vi "Count Encoder.vi"(0 "Encoder A Prev. Signal In":bool, 5 "Encoder B Prev. Signal In":bool, 7 "Encoder A Signal In":bool, 9 "Encoder B Signal In":bool, 11 "Encoder Count In":i64) -> (15 "Encoder Count Out":i64)   [LabVIEW 2016]
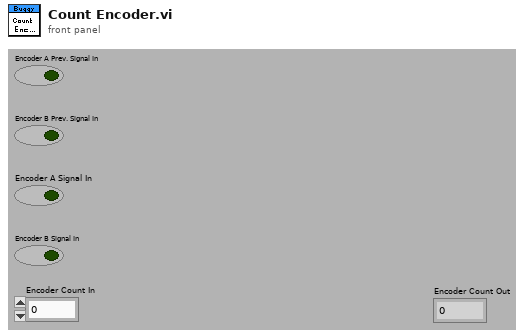
[diagram p1: front panel]
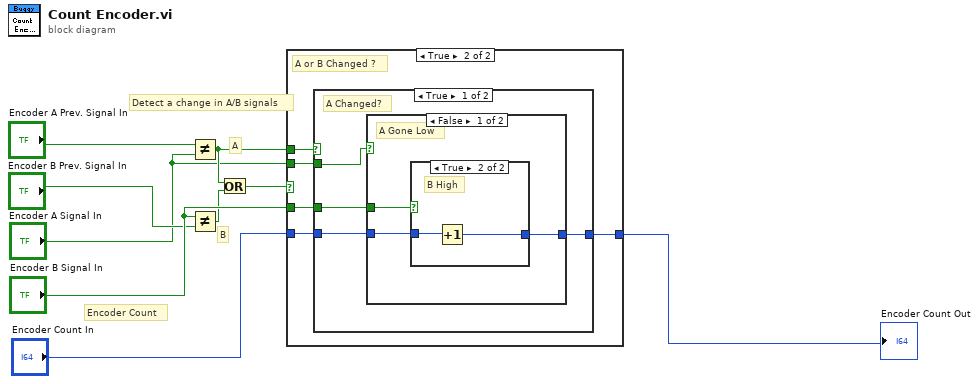
[diagram p0: block diagram]
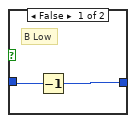
[diagram p3: hidden frame]
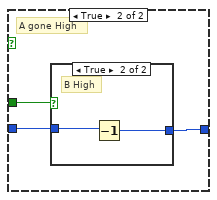
[diagram p4: hidden frame]
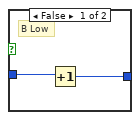
[diagram p5: hidden frame]
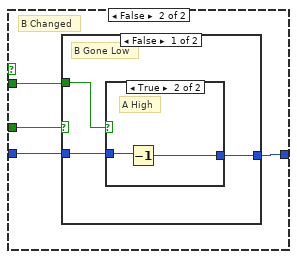
[diagram p6: hidden frame]
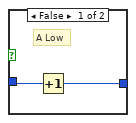
[diagram p7: hidden frame]
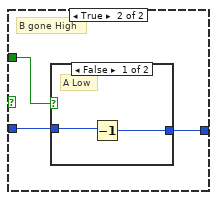
[diagram p8: hidden frame]
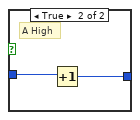
[diagram p9: hidden frame]
diagram:
  # "Encoder Count"
  # "B"
  # "A"
  # "Detect a change in A/B signals"
  n1 = Not Equal?(x="Encoder A Prev. Signal In", y="Encoder A Signal In") -> (x != y?=w8:bool)
  n2 = Not Equal?(x="Encoder B Signal In", y="Encoder B Prev. Signal In") -> (x != y?=w6:bool)
  n3 = Or(x=w8, y=w6) -> (x .or. y?=w5:bool)
  n4 = case shown="True" w5 {
    tunnel: w8 -> [_ w15]
    tunnel: "Encoder Count In" -> [w10 w14]
    tunnel: "Encoder A Signal In" -> [_ w13]
    tunnel: "Encoder B Signal In" -> [_ w12]
    tunnel: [w10 w11] -> w7
    frame False {
      # "A or B not changed Keep Existing encoder count"
    }
    frame True {
      # "A or B Changed ?"
      n5 = case shown="True" w15 {
        tunnel: w14 -> [w19 w37]
        tunnel: w12 -> [w18 w36]
        tunnel: w13 -> [w17 w35]
        tunnel: [w16 w34] -> w11
        frame True {
          # "A Changed?"
          n6 = case shown="False" w17 {
            tunnel: w19 -> [w21 w28]
            tunnel: w18 -> [w22 w29]
            tunnel: [w20 w27] -> w16
            frame False {
              # "A Gone Low"
              n7 = case shown="True" w22 {
                tunnel: w21 -> [w24 w26]
                tunnel: [w23 w25] -> w20
                frame False {
                  # "B Low"
                  n8 = Decrement(x=w24) -> (x-1=w23:i64)
                }
                frame True {
                  # "B High"
                  n9 = Increment(x=w26) -> (x+1=w25:i64)
                }
              }
            }
            frame True {
              # "A gone High"
              n10 = case shown="True" w29 {
                tunnel: w28 -> [w30 w33]
                tunnel: [w31 w32] -> w27
                frame False {
                  # "B Low"
                  n11 = Increment(x=w30) -> (x+1=w31:i64)
                }
                frame True {
                  # "B High"
                  n12 = Decrement(x=w33) -> (x-1=w32:i64)
                }
              }
            }
          }
        }
        frame False {
          # "B Changed"
          n13 = case shown="False" w36 {
            tunnel: w37 -> [w40 w47]
            tunnel: [w39 w46] -> w34
            tunnel: w35 -> [w38 w45]
            frame False {
              # "B Gone Low"
              n14 = case shown="True" w38 {
                tunnel: w40 -> [w42 w44]
                tunnel: [w41 w43] -> w39
                frame False {
                  # "A Low"
                  n15 = Increment(x=w42) -> (x+1=w41:i64)
                }
                frame True {
                  # "A High"
                  n16 = Decrement(x=w44) -> (x-1=w43:i64)
                }
              }
            }
            frame True {
              # "B gone High"
              n17 = case shown="False" w45 {
                tunnel: w47 -> [w48 w51]
                tunnel: [w49 w50] -> w46
                frame False {
                  # "A Low"
                  n18 = Decrement(x=w48) -> (x-1=w49:i64)
                }
                frame True {
                  # "A High"
                  n19 = Increment(x=w51) -> (x+1=w50:i64)
                }
              }
            }
          }
        }
      }
    }
  }
  "Encoder Count Out" <- w7
